vi "ExecutableInstance.vi"(11 "error in (no error)":errorcluster) -> (15 "error out":errorcluster)   [LabVIEW 2016, in "Drona Test.lvlib"]
uses:
  Drona Test.lvlib
  main/apis/Setup/GetVI/GetVIByName.vi
  main/apis/Stimulus/VI/MakeVIFrontMost.vi
  <vilib>/addons/_JKI Toolkits/Caraya/classes/Assert/Assert Not Error.vi
  main/Drona.lvlib
  main/apis/Setup/GetVI/GetVI.lvlib
  <vilib>/addons/_JKI Toolkits/Caraya/classes/Assert/Assert.lvclass
  <vilib>/addons/_JKI Toolkits/Caraya/classes/Test/Test.lvclass
  main/apis/Stimulus/VI/VI.lvlib
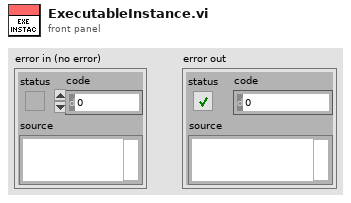
[diagram p1: front panel]
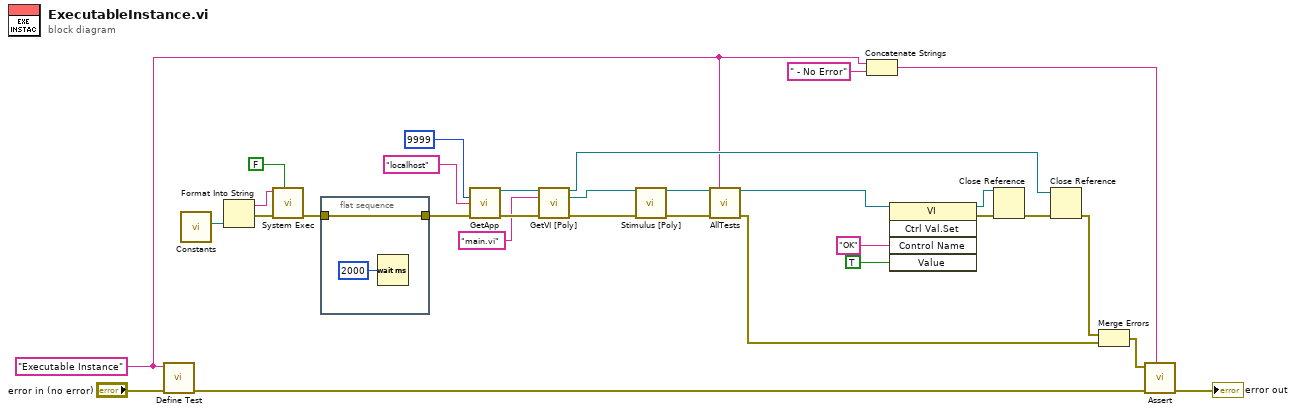
[diagram p0: block diagram]
diagram:
  w3 = "Executable Instance" ("Label (VI Title)")
  n1 = call <vilib>:"Define Test.vi"("error in (no error)"="error in (no error)", "Label (VI Title)"=w3) -> ("error out"=w28:errorcluster)  [unwired: 9 in]
  n2 = call "Constants.vi"() -> ("HelperExecutable path"=w4:path)  [unwired: 9 in, 2 out]
  n3 = Format Into String(w4) -> (resulting string=w18:string, error out=w19:errorcluster)  [unwired: 3 in]
  n4 = call <vilib>:"System Exec.vi"("wait until completion? (T)"=FALSE, "error in (no error)"=w19, "command line"=w18) -> ("error out"=w9:errorcluster)  [unwired: 5 in, 3 out]
  n5 = flat-sequence {
    tunnel: [w33] -> w10
    tunnel: w9 -> [w33]
    frame #0 {
      n6 = Wait (ms)(milliseconds to wait=u32 2000) -> ()  [unwired: 1 out]
    }
  }
  n7 = call "GetApp.vi"("Port(0:Ignored)"=u16 9999, "Service Name (\"\":localhost)"="localhost" ("Project Name (\"\": ThisApplication)"), "error in (no error)"=w10) -> ("Application Ref"=w23:refnum<vi>, "error out"=w22:errorcluster)  [unwired: 11 in]
  n8 = call-poly "GetVI [Poly].vi"("Application Ref in"=w23, "VI Name"="main.vi", "error in (no error)"=w22) -> ("Application Ref out"=w24:refnum<vi>, "VI Reference"=w8:refnum<vi>, "error out"=w6:errorcluster)  [unwired: 10 in]
  n9 = call-poly "Stimulus [Poly].vi"("VI Reference In"=w8, "error in"=w6) -> ("VI Reference Out"=w7:refnum<vi>, "error out"=w5:errorcluster)  [unwired: 12 in]
  n10 = call "AllTests.vi"("VI in"=w7, "Label"=w3, "error in (no error)"=w5) -> ("VI out"=w25:refnum<vi>, "error out"=w2:errorcluster)  [unwired: 11 in]
  n11 = Concatenate Strings(w3, " - No Error" ("Label (VI Title)")) -> (w26:string)
  n12 = invoke class="VI" method="Ctrl Val.Set"(reference=w25, "Control Name"="OK", "Value"=TRUE) -> (reference out=w15:refnum<vi>, error out=w16:errorcluster)  [unwired: 2 in, 3 out]
  n13 = Close Reference(reference=w15, error in (no error)=w16) -> (error out=w12:errorcluster)
  n14 = Close Reference(reference=w24, error in (no error)=w12) -> (error out=w1:errorcluster)
  n15 = Merge Errors(w1, w2) -> (w31:errorcluster)
  n16 = call-poly <vilib>:"Assert.vi"("Label"=w26, "error in (no error)"=w28, "Not Error?"=w31) -> ("error out"=→"error out":errorcluster)  [unwired: 8 in]
